vi "citTemplate.writeQueueWithAckOrig.vi"(0 "timeout ms (-1)":i32=-1, 1 "High priority (F)":bool, 2 "instance (0)":i32, 3 "timeout error code (5003)":i32=5003, 5 "event in":variant, 9 "(flatten) data in":string, 11 "error in (no error)":errorcluster) -> (6 "dup of event":variant, 10 "notification data":string, 15 "error out":errorcluster)   [LabVIEW 2015]
uses:
  citTemplate.eventQueue.ctl
  citTemplate.notifierData.ctl
  citTemplate.notifierHandle.ctl
  citTemplate.queueData.ctl
panel:
  # "REENTRANT !!!!"
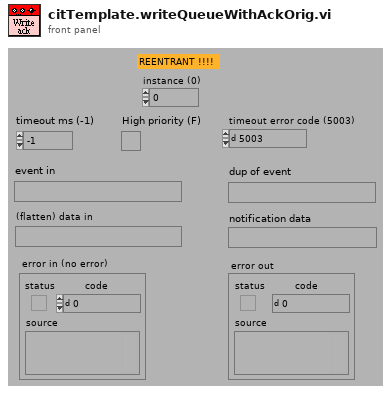
[diagram p1: front panel]
types:
  T1 = typedef "citTemplate.queueData.ctl" = cluster{"event index":u32, "(flatten) data in":string, "notifierHandle":T2}
  T2 = typedef "citTemplate.notifierHandle.ctl" = refnum<notifier>
  T3 = typedef "citTemplate.eventQueue.ctl" = enum16{"create queue", "get queue handle(s)", "destroy queue"}
  T4 = typedef "citTemplate.notifierData.ctl" = cluster{"notification data":string, "error":errorcluster}
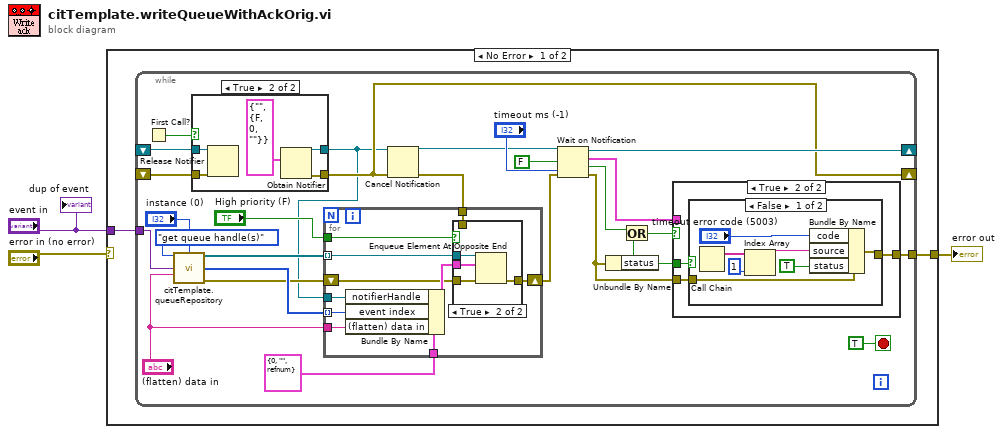
[diagram p0: block diagram]
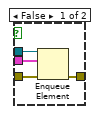
[diagram p2: hidden frame]
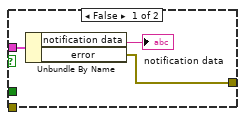
[diagram p3: hidden frame]
diagram:
  n1 = case shown="No Error" "error in (no error)" {
    selector: "error in (no error)" -> [_ w72]
    tunnel: [w5 w72] -> w3
    tunnel: "event in" -> [w4 _]
    frame No Error {
      n2 = while {
        shift-right: [w25] -> _
        shift-left: _ -> [w31]
        shift-right: [w18] -> _
        shift-left: _ -> [w30]
        tunnel: [w28] -> w5
        tunnel: w4 -> [w14]
        stop <- TRUE stop-if-true
        n3 = First Call?() -> (First Call?: T/F=w32:bool)
        n4 = call "citTemplate.queueRepository.vi"("mode (get queue handle)"=citTemplate.eventQueue."get queue handle(s)" ("mode (write event)"), "instance (0)"="instance (0)", "event in"=w14, "(flatten) data in"="(flatten) data in") -> ("queueHandle(s) out"=w16:refnum<queue>[], "eventIndex(s)"=w11:u32[], "error out"=w10:errorcluster)  [unwired: 4 in, 5 out]
        n5 = case shown="True" w32 {
          tunnel: [w66 w71] -> w6
          tunnel: [w65 w70] -> w18
          tunnel: w31 -> [w66 w69]
          tunnel: w30 -> [w65 w68]
          frame False {
          }
          frame True {
            n6 = Release Notifier(notifier=w69, error in (no error)=w68) -> ()  [unwired: 4 out]
            n7 = Obtain Notifier(notification data type=T4 {"notification data"="", "error"={"status"=FALSE, "code"=0, "source"=""}} ("notifierData")) -> (notifier out=w71:refnum<notifier>, error out=w70:errorcluster)  [unwired: 2 in, 2 out]
          }
        }
        n8 = Cancel Notification(0:w6, 3:w18) -> (8:w17:refnum<notifier>, 11:w12:errorcluster)  [unwired: 1 out]
        n9 = for {
          tunnel: w16 -> [w42] mode=indexing
          tunnel: "(flatten) data in" -> [w40]
          tunnel: "High priority (F)" -> [w39]
          tunnel: w6 -> [w38]
          tunnel: w12 -> [w37]
          tunnel: w11 -> [w36] mode=indexing
          shift-right: [w34] -> w9
          shift-left: w10 -> [w35]
          tunnel: T1 {"event index"=0, "(flatten) data in"="", "notifierHandle"=refnum} ("queueData") -> [w33]
          n10 = Bundle By Name(cluster=w33, "notifierHandle"=w38, "event index"=w36, "(flatten) data in"=w40) -> (w41:T1)
          n11 = case shown="True" w39 {
            tunnel: w42 -> [w46 w50]
            tunnel: w35 -> [w45 w49]
            tunnel: [w44 w48] -> w34
            tunnel: w41 -> [w43 w47]
            tunnel: w37 -> [_ _]
            frame False {
              n12 = Enqueue Element(queue=w46, element=w43, error in (no error)=w45) -> (error out=w44:errorcluster)  [unwired: 3 out]
            }
            frame True {
              n13 = Enqueue Element At Opposite End(queue=w50, element=w47, error in (no error)=w49) -> (error out=w48:errorcluster)  [unwired: 3 out]
            }
          }
        }
        n14 = Wait on Notification(notifier=w17, ignore previous (F)=FALSE ("ignore previous (T)"), timeout in ms (-1)="timeout ms (-1)", error in (no error)=w9) -> (notifier out=w25:refnum<notifier>, notification=w24:T4, timed out?=w21:bool, error out=w22:errorcluster)
        n15 = Unbundle By Name(w22) -> ("status"=w20:bool)
        n16 = Or(x=w21, y=w20) -> (x .or. y?=w23:bool)
        n17 = case shown="True" w23 {
          tunnel: w24 -> [w53 _]
          tunnel: [w52 w54] -> w28
          tunnel: w22 -> [_ w56]
          tunnel: w20 -> [_ w55]
          frame False {
            n18 = Unbundle By Name(w53) -> ("notification data"=→"notification data":string, "error"=w52:errorcluster)
          }
          frame True {
            n19 = case shown="False" w55 {
              tunnel: w56 -> [w63 w64]
              tunnel: [w62 w64] -> w54
              frame False {
                n20 = Call Chain() -> (call chain=w59:string[])
                n21 = Index Array(array=w59, index=1) -> (element=w58:string)
                n22 = Bundle By Name(cluster=w63, "code"="timeout error code (5003)", "source"=w58, "status"=TRUE) -> (w62:errorcluster)
              }
              frame True {
              }
            }
          }
        }
      }
    }
    frame Error {
    }
  }
  "error out" <- w3
  "dup of event" <- "event in"
